vi "Configure OutPut Timer State and Delay.vi"(8 "error in":errorcluster, 9 "Time Delay(S)":dbl=1.0 min=1.0 max=86400.0, 10 "State":bool, 11 "VISA resource name":refnum<visa-resource-name>) -> (0 "error out":errorcluster, 3 "VISA resource name out":refnum<visa-resource-name>)   [LabVIEW 2018, in "IT-M3100.lvlib"]
doc: "This command sets the timing function status and time.\n<b>State</b>\n0:Close the State\n1:Open the state\n<b>Time Delay(S)</b>\n1-86400"
uses:
  IT-M3100.lvlib
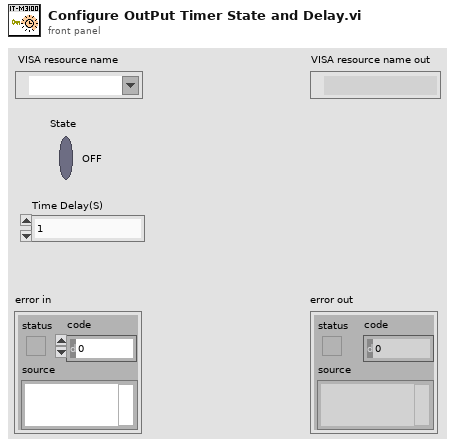
[diagram p1: front panel]
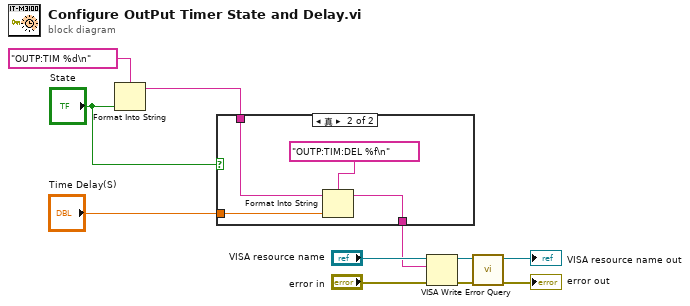
[diagram p0: block diagram]
diagram:
  n1 = Format Into String(format string="OUTP:TIM %d\n", "State") -> (resulting string=w4:string)  [unwired: 2 in, 1 out]
  n2 = case shown="真" "State" {
    tunnel: w4 -> [w12 w15]
    tunnel: "Time Delay(S)" -> [_ w14]
    tunnel: [w12 w13] -> w1
    frame False {
    }
    frame True {
      n3 = Format Into String(format string="OUTP:TIM:DEL %f\n", initial string=w15, w14) -> (resulting string=w13:string)  [unwired: 1 in, 1 out]
    }
  }
  n4 = VISA Write(VISA resource name="VISA resource name", write buffer=w1, error in (no error)="error in") -> (VISA resource name out=w8:refnum<visa-resource-name>, error out=w9:errorcluster)  [unwired: 1 out]
  n5 = call "Error Query.vi"("error in"=w9, "VISA resource name"=w8) -> ("error out"=→"error out":errorcluster, "VISA resource name out"=→"VISA resource name out":refnum<visa-resource-name>)  [unwired: 6 in, 2 out]
